vi "test_Bitfile Reload_Scalar to Static Scalar Data Type Change.vi"(8 "error in (no error)":errorcluster, 11 "TestCase in":refnum<class "FPGA Addon Bitfile Reload Unit Tests.lvclass">=refnum) -> (0 "error out":errorcluster, 3 "TestCase out":refnum<class "FPGA Addon Bitfile Reload Unit Tests.lvclass">)   [LabVIEW 2026, in "FPGA Addon Bitfile Reload Unit Tests.lvclass"]
uses:
  FPGA Addon Bitfile Reload Unit Tests.lvclass
  FPGA Addon Test Class/FPGA Addon Test Class.lvclass
  APIs/Scripting API/Scripting API.lvlib
  Addon/Addon System Explorer/FPGA Addon System Explorer.lvlib
  APIs/Scripting API/TypeDefs/Output Scalar Data.ctl
  Addon/Addon Shared/SubVIs/Constants.vi
  Addon/Addon Shared/FPGA Addon Shared.lvlib
  APIs/Scripting API/Public/Bitfile Resources/Import Bitfile Scalars (Instances)/Import Scalars - all.vi
  Addon/Addon Shared/Types/FPGA Addon Data Type.ctl
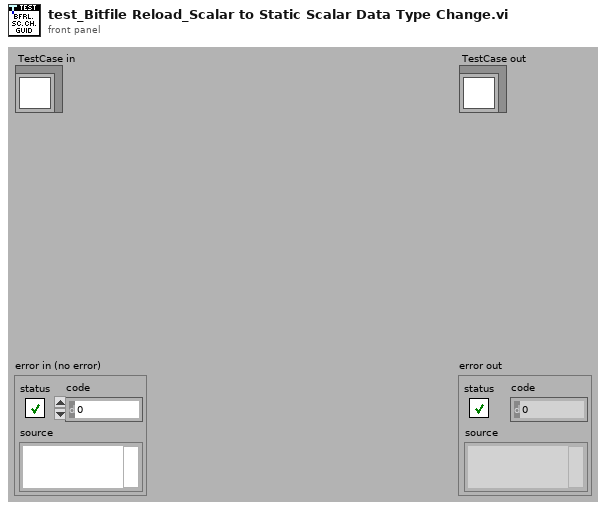
[diagram p1: front panel]
types:
  T1 = typedef "Scripting API.lvlib/Output Scalar Data.ctl" = cluster{"Bitfile Name":string, "SysDef Channel Name":string, "Imported":bool, "Data Type":T2}
  T2 = typedef "FPGA Addon Shared.lvlib/FPGA Addon Data Type.ctl" = enum8{"<Null>", "I8", "I16", "I32", "I64", "U8", "U16", "U32", "U64", "SGL", "Boolean", "Analog PWM In Settings", "Analog PWM In", "Digital PWM In Settings", "Digital PWM In", "Digital PWM Out", "Sine Out", "FXP", "FXP+/-24.5", "FXP+/-16.5", "FXP+/-32.8", "FXP+/-64.32", "FXP+/-16.7", "FXP+/-20.5", "FXP+/-27.5", "FXP+/-32.16", "FXP+16.3", "FXP+18.3", "Digital Static In", "Digital Static Out", "Digital Static In Settings", "Digital WSS Out", "Quad Encoder Settings", "Quad Encoder In", "Group"}
  T3 = typedef "Custom Device API.lvlib/Custom Device Item Ref.ctl" = u64
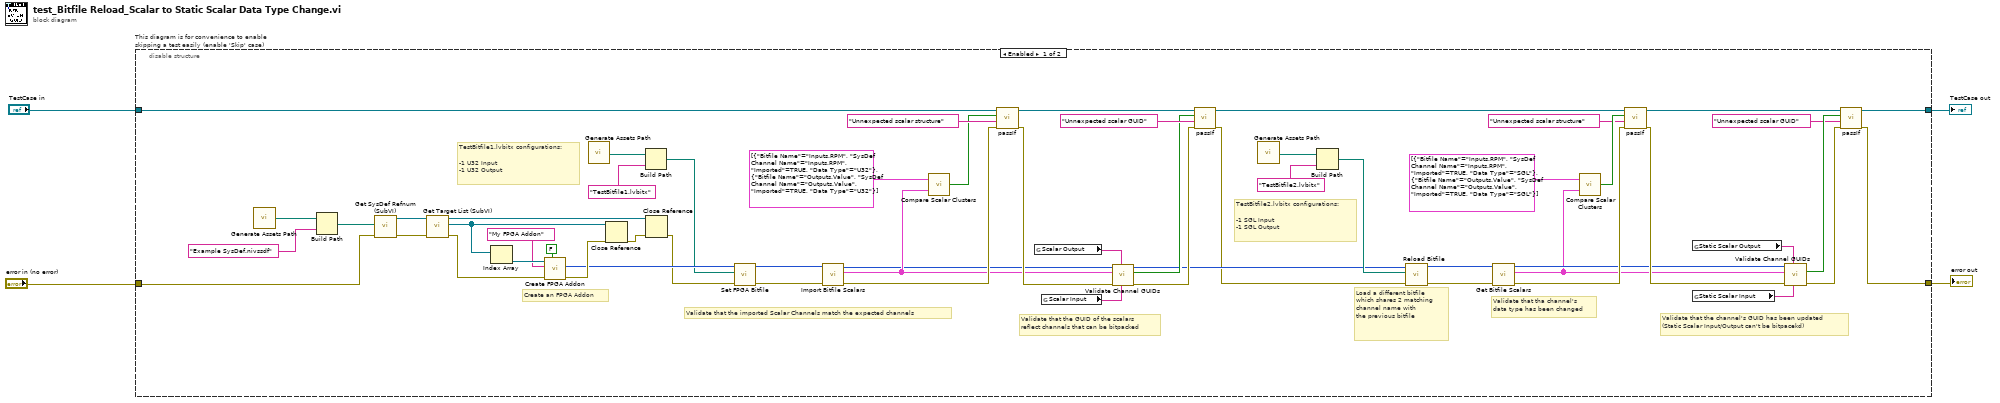
[diagram p0: block diagram]
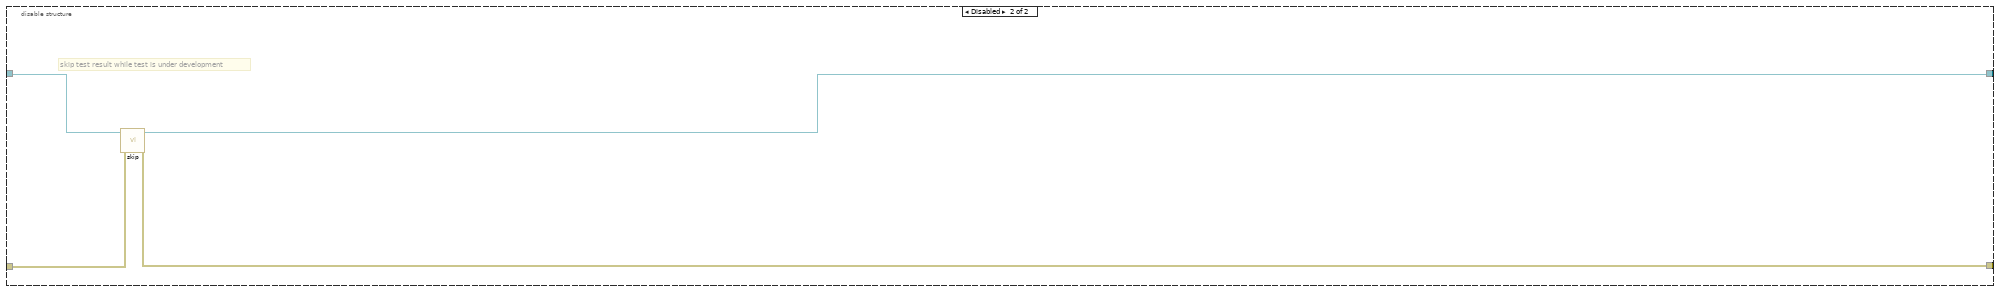
[diagram p2: hidden frame]
diagram:
  n1 = disable-structure "This diagram is for convenience to enable skipping a test easily (enable 'Skip' case)" shown="Enabled" {
    disable-tunnel: "TestCase in" -> [w31 w66]
    disable-tunnel: [w5 w64] -> w1
    disable-tunnel: [w6 w65] -> w3
    disable-tunnel: "error in (no error)" -> [w30 w63]
    frame Enabled {
      # "Validate that the GUID of the scalars\nreflect channels that can be bitpacked"
      # "Validate that the channel's GUID has been updated\n(Static Scalar Input/Output can't be bitpacekd)"
      # "TestBitfile2.lvbitx configurations:\n\n-1 SGL Input\n-1 SGL Output"
      # "TestBitfile1.lvbitx configurations:\n\n-1 U32 Input\n-1 U32 Output"
      # "Validate that tha channel's \ndata type has been changed"
      # "Load a different bitfile\nwhich shares 2 matching\nchannel name with \nthe previous bitfile"
      # "Validate that the imported Scalar Channels match the expected channels"
      # "Create an FPGA Addon"
      n2 = call "Generate Assets Path.vi"() -> ("Assets path"=w42:path)
      n3 = Build Path(base path=w42, name or relative path="Example SysDef.nivssdf") -> (appended path=w61:path)
      n4 = call "Get SysDef Refnum (SubVI).vi"("error in (no error)"=w30, "System Definition path"=w61) -> ("error out"=w57:errorcluster, "NationalInstruments.VeriStand.SystemDefinitionAPI.SystemDefinition"=w60:refnum<k39>)  [unwired: 8 in]
      n5 = call "Get Target List (SubVI).vi"("error in (no error)"=w57, "NationalInstruments.VeriStand.SystemDefinitionAPI.SystemDefinition"=w60) -> ("error out"=w56:errorcluster, "Target List Refnums"=w55:refnum<k39>[], "NationalInstruments.VeriStand.SystemDefinitionAPI.SystemDefinition"=w54:refnum<k39>)  [unwired: 7 in]
      n6 = Index Array(array=w55) -> (element=w59:refnum<k39>)  [unwired: 1 in]
      n7 = call "Create FPGA Addon.vi"("group scalars"=FALSE, "error in"=w56, "FPGA addon name"="My FPGA Addon", "NationalInstruments.VeriStand.SystemDefinitionAPI.Target"=w59) -> ("error out"=w52:errorcluster, "FPGA addon refnum"=w50:T3)  [unwired: 5 in, 1 out]
      n8 = call "Generate Assets Path.vi"() -> ("Assets path"=w41:path)
      n9 = Close Reference(reference=w55, error in (no error)=w52) -> (error out=w53:errorcluster)
      n10 = Build Path(base path=w41, name or relative path="TestBitfile1.lvbitx") -> (appended path=w47:path)
      n11 = Close Reference(reference=w54, error in (no error)=w53) -> (error out=w49:errorcluster)
      n12 = call "Set FPGA Bitfile.vi"("error in"=w49, "FPGA bitfile path"=w47, "FPGA addon refnum in"=w50) -> ("error out"=w46:errorcluster, "FPGA addon refnum out"=w45:T3)  [unwired: 7 in]
      n13 = call-poly "Import Bitfile Scalars.vi"("error in"=w46, "FPGA addon refnum in"=w45) -> ("error out"=w44:errorcluster, "imported bitfile scalars out"=w21:T1[], "FPGA addon refnum out"=w20:T3)  [unwired: 7 in]
      n14 = call "Compare Scalar Clusters.vi"("Target bitfile scalars in"=w21, "Reference bitfile scalars in"=T1[] [{"Bitfile Name"="Inputs.RPM", "SysDef Channel Name"="Inputs.RPM", "Imported"=TRUE, "Data Type"=enum."U32"}, {"Bitfile Name"="Outputs.Value", "SysDef Channel Name"="Outputs.Value", "Imported"=TRUE, "Data Type"=enum."U32"}] ("imported bitfile scalars out")) -> ("Equal ?"=w40:bool)
      n15 = call-dynamic "passIf.vi"("error in (no error)"=w44, "message (\"\")"="Unnexpected scalar structure" ("message (\"\")"), "pass"=w40, "TestCase in"=w31) -> ("error out"=w27:errorcluster, "TestCase out"=w26:refnum<class "FPGA Addon Bitfile Reload Unit Tests.lvclass">)  [unwired: 6 in]
      n16 = global read "Constants.vi" "Scalar Output"() -> (w23:string)
      n17 = global read "Constants.vi" "Scalar Input"() -> (w22:string)
      n18 = call "Validate Channel GUIDs.vi"("input GUID"=w22, "output GUID"=w23, "error in (no error)"=w27, "imported bitfile scalars in"=w21, "FPGA addon refnum in"=w20) -> ("error out"=w24:errorcluster, "valid GUIDs?"=w19:bool, "FPGA addon refnum out"=w18:T3)  [unwired: 4 in]
      n19 = call-dynamic "passIf.vi"("error in (no error)"=w24, "message (\"\")"="Unnexpected scalar GUID" ("message (\"\")"), "pass"=w19, "TestCase in"=w26) -> ("error out"=w17:errorcluster, "TestCase out"=w16:refnum<class "FPGA Addon Bitfile Reload Unit Tests.lvclass">)  [unwired: 6 in]
      n20 = call "Generate Assets Path.vi"() -> ("Assets path"=w38:path)
      n21 = Build Path(base path=w38, name or relative path="TestBitfile2.lvbitx") -> (appended path=w37:path)
      n22 = call "Reload Bitfile.vi"("error in (no error)"=w17, "NewVal"=w37, "Item Ref in"=w18) -> ("error out"=w36:errorcluster, "Section Ref out"=w35:T3)  [unwired: 7 in]
      n23 = call "Get Bitfile Scalars.vi"("error in"=w36, "FPGA addon refnum in"=w35) -> ("error out"=w34:errorcluster, "bitfile scalars out"=w11:T1[], "FPGA addon refnum out"=w12:T3)  [unwired: 7 in]
      n24 = call "Compare Scalar Clusters.vi"("Target bitfile scalars in"=w11, "Reference bitfile scalars in"=T1[] [{"Bitfile Name"="Inputs.RPM", "SysDef Channel Name"="Inputs.RPM", "Imported"=TRUE, "Data Type"=enum."SGL"}, {"Bitfile Name"="Outputs.Value", "SysDef Channel Name"="Outputs.Value", "Imported"=TRUE, "Data Type"=enum."SGL"}] ("bitfile scalars out")) -> ("Equal ?"=w33:bool)
      n25 = call-dynamic "passIf.vi"("error in (no error)"=w34, "message (\"\")"="Unnexpected scalar structure" ("message (\"\")"), "pass"=w33, "TestCase in"=w16) -> ("error out"=w13:errorcluster, "TestCase out"=w10:refnum<class "FPGA Addon Bitfile Reload Unit Tests.lvclass">)  [unwired: 6 in]
      n26 = global read "Constants.vi" "Static Scalar Output"() -> (w15:string)
      n27 = global read "Constants.vi" "Static Scalar Input"() -> (w14:string)
      n28 = call "Validate Channel GUIDs.vi"("input GUID"=w14, "output GUID"=w15, "error in (no error)"=w13, "imported bitfile scalars in"=w11, "FPGA addon refnum in"=w12) -> ("error out"=w9:errorcluster, "valid GUIDs?"=w8:bool)  [unwired: 4 in, 1 out]
      n29 = call-dynamic "passIf.vi"("error in (no error)"=w9, "message (\"\")"="Unnexpected scalar GUID" ("message (\"\")"), "pass"=w8, "TestCase in"=w10) -> ("error out"=w6:errorcluster, "TestCase out"=w5:refnum<class "FPGA Addon Bitfile Reload Unit Tests.lvclass">)  [unwired: 6 in]
    }
    frame Disabled {
      # "skip test result while test is under development"
      n30 = call <vilib>:"skip.vi"("error in (no error)"=w63, "TestCase in"=w66) -> ("error out"=w65:errorcluster, "TestCase out"=w64:refnum<class "FPGA Addon Bitfile Reload Unit Tests.lvclass">)  [unwired: 8 in]
    }
  }
  "error out" <- w3
  "TestCase out" <- w1
